vi "oath2_auth_url.vi"   [LabVIEW 2015, in "lv-dropbox.lvlib"]
uses:
  lv-dropbox.lvlib
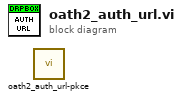
[diagram p0: block diagram]
diagram:
  n1 = call "oath2_auth_url-pkce.vi"() -> ()  [unwired: 10 in, 2 out]
